vi "Sequencer.201812.vi"() -> ()   [LabVIEW 2014]
uses:
  <vilib>/gmath/statdist.llb/Poisson Random.vi
  <vilib>/Analysis/NI_AALPro.lvlib
  <vilib>/gmath/NI_Gmath.lvlib
panel:
  in  "Ion":bool
  in  "Protect":bool
  in  "Experiment":bool
  in  "Pumping":bool
  in  "Detection":bool
  in  "Cooling":bool
  out "History":variant
  in  "Count or State":i16(ring) items=["Count", "State"]
  in  "Channel":string(combo)="c1+c2+c3+c4"
  in  "Device":string(combo)="PMT"
  in  ">":dbl=1.0
  in  "Fit":bool
  out "Peak":u32
  out "Histogram":cluster{"Axis":dbl[], "Histogram":i32[]}(graph)
  in  "Data Chapter":i16(ring) items=["All", "Detection[2]"]
  out "Average Plot":cluster{dbl, dbl}(graph)
  in  "Clear":bool
  in  "Sweep":bool
  in  "Data":bool
  out "data file":string
  in  "Sequence":string
  in  "Chapter (us)":string
  in  "Sequence File":path=path "E:/Data/Sequence/Cooling.seq"
  in  "Repeats":u32=100
  in  "Compile":bool
  in  "Send":bool
  in  "Port":refnum<visa-resource-name>="COM5"
  in  "Trigger":bool
  in  "Save":bool
  out "Item Function":refnum<vi>
  in  "Set":bool
  in  "Item":string(combo)="Time"
  out "SequenceNames":string[](array[string])
  in  "Parameter":u16(ring) items=["Cooling", "Pumping", "AWG", "Horn", "Detection[0]", "Detection[1]", "Detection[2]", "Zero"]
  in  "Scan":bool
  out "Value":dbl=1.0 format="%.4f"
  in  "Step":dbl=1.0 format="%.4f"
  in  "End":dbl=1.0 format="%.3f"
  in  "Start":dbl=1.0 format="%.3f"
  out "Counts":u32[](array[numeric])
  out "CompiledSequence":string="#DopplerCooling\r\n0.9 10100000 00000000 00000000\r\n\r\n#Pump\r\n0.3 01000000 00000000 00000000\r\n\r\n#Pulsed\r\n0.2 00100000 00000000 00000000\r\n0.4 00000100 00000000 00000000\r\n0.2 00000000 10000000 00000000\r\n0.2 01000000 00000000 01000000\n"
  out "ChapterNames":string[](array[string])
  out "ChapterPositions":u32[](array[numeric])
  out "Durations Backup":dbl[](array[numeric])
  out "Durations":dbl[](array[numeric])
  in  "Period (ns)":dbl=5.0
  out "States":string[](array[string])
  in  "Sequencer":bool
  out "Clock":string
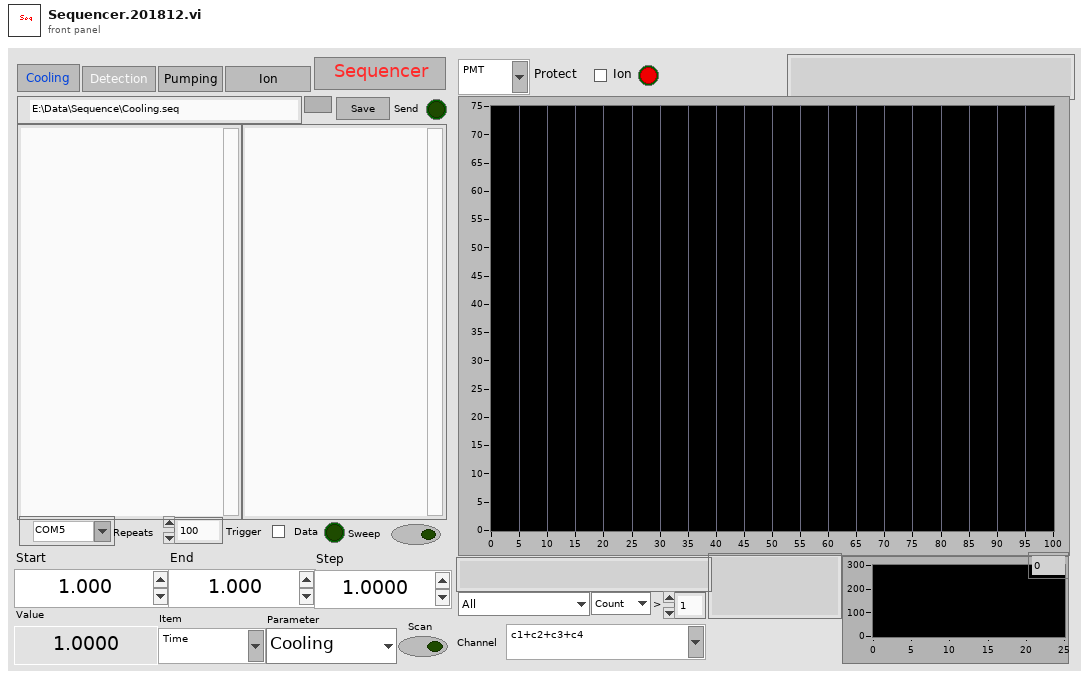
[diagram p1: front panel]
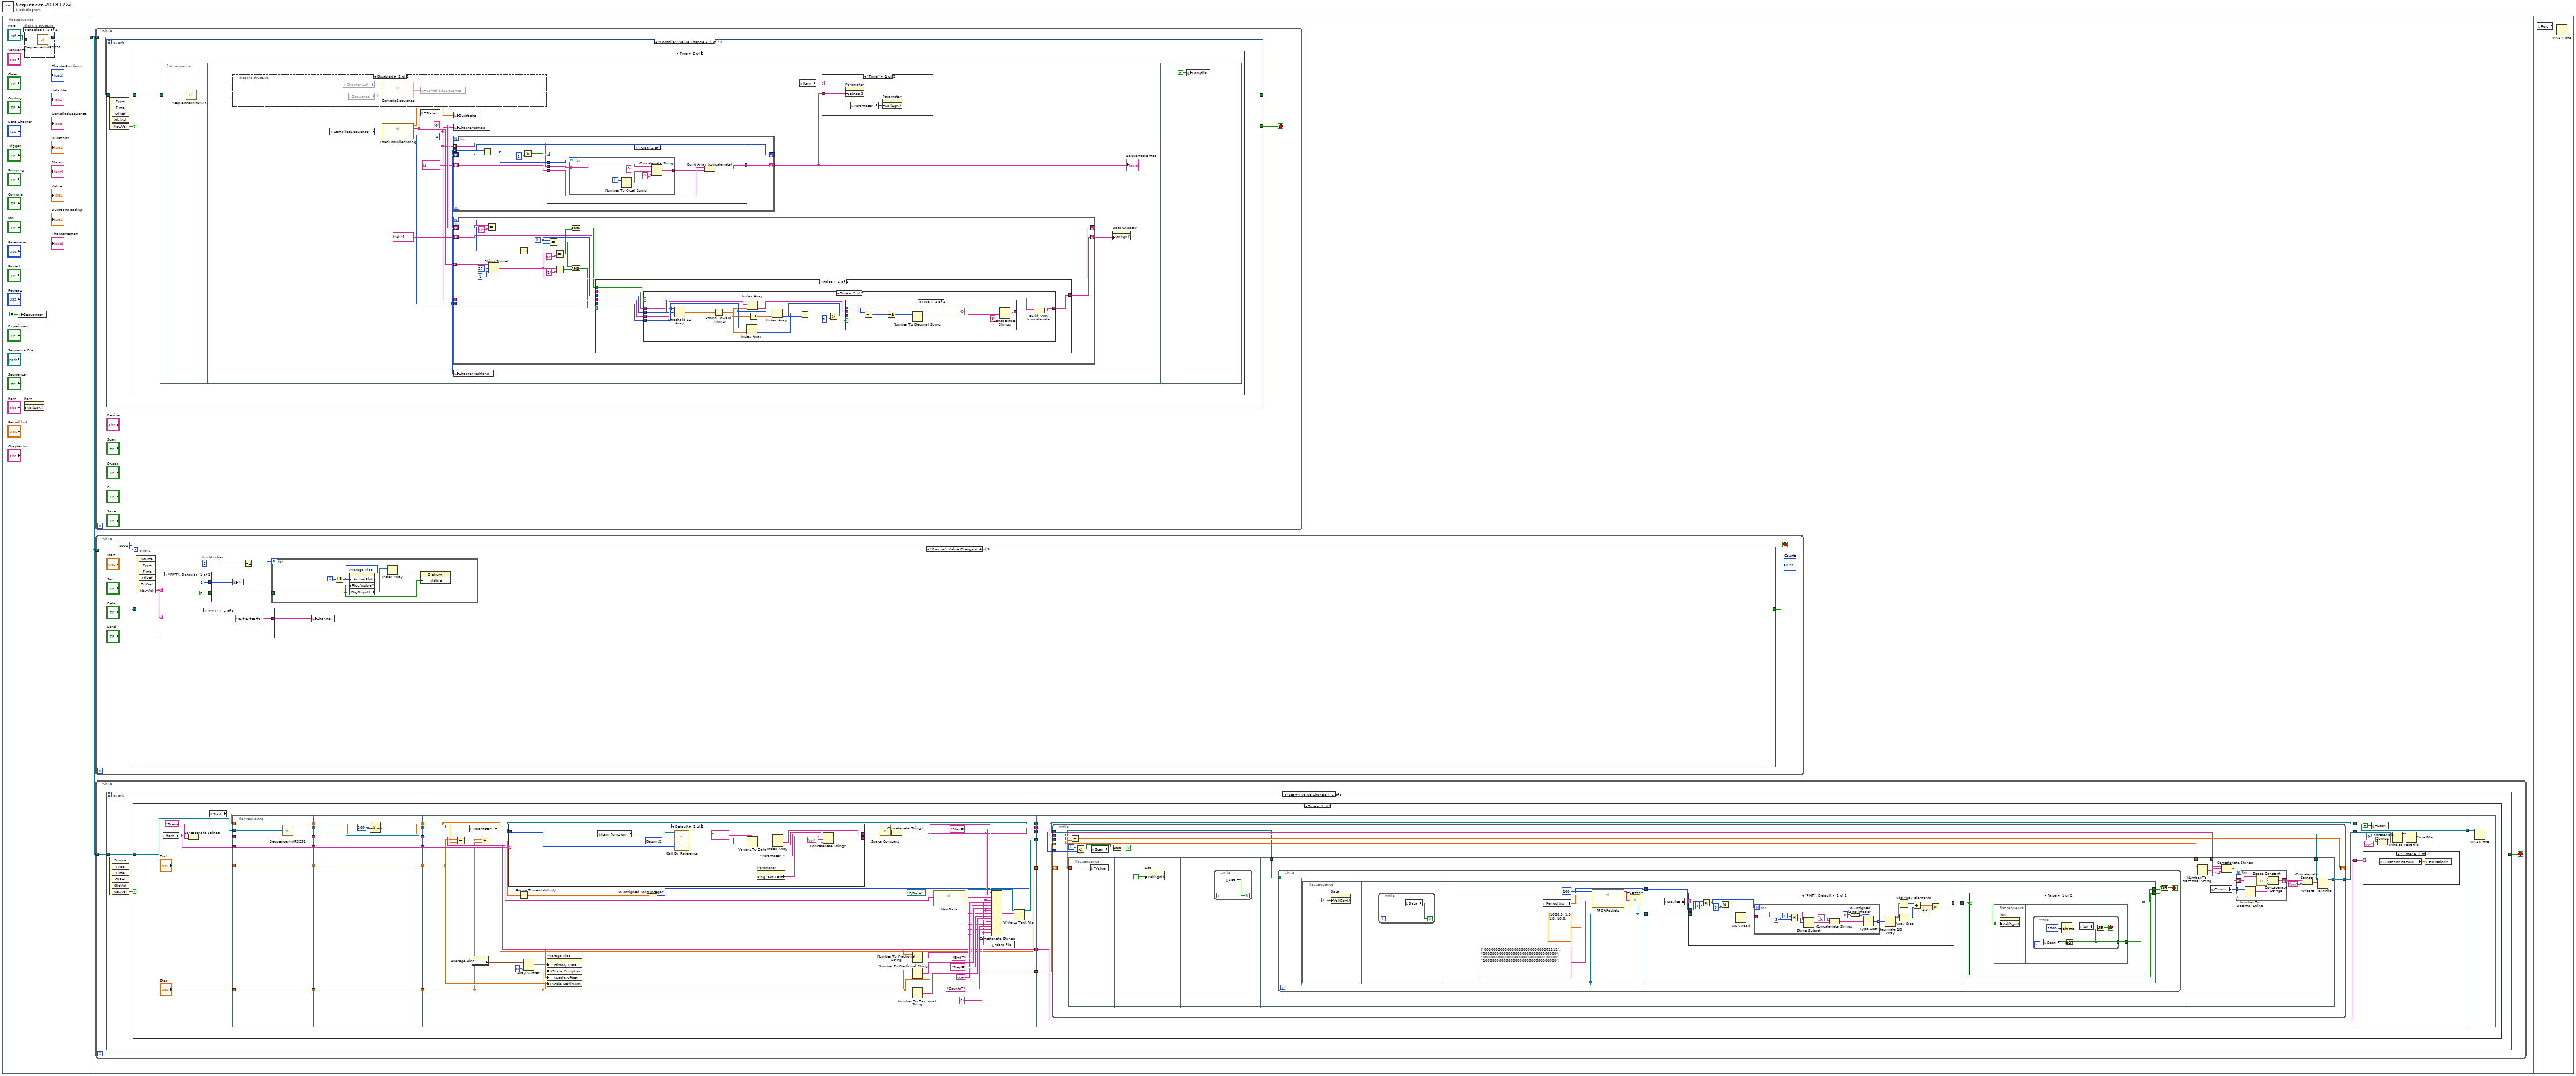
[diagram p0: block diagram]
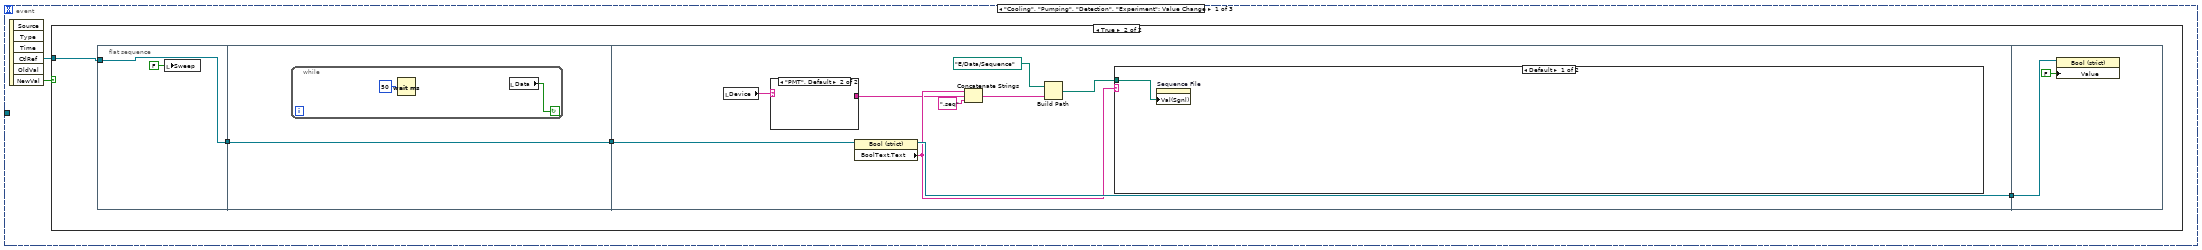
[diagram p3: hidden frame]
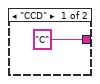
[diagram p5: hidden frame]
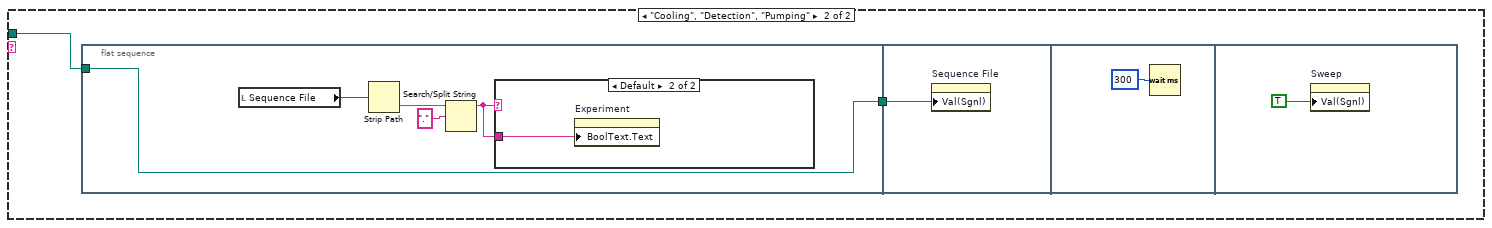
[diagram p6: hidden frame]
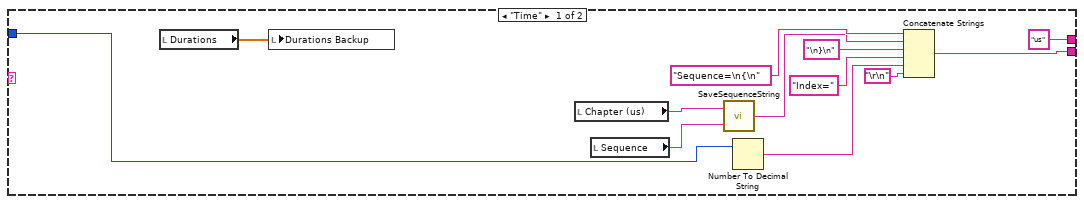
[diagram p8: hidden frame]
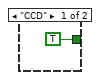
[diagram p9: hidden frame]
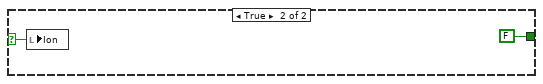
[diagram p10: hidden frame]
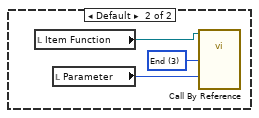
[diagram p11: hidden frame]
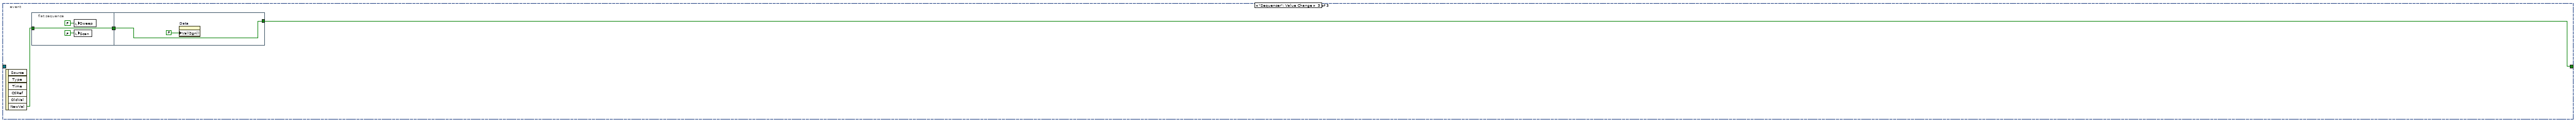
[diagram p13: hidden frame]
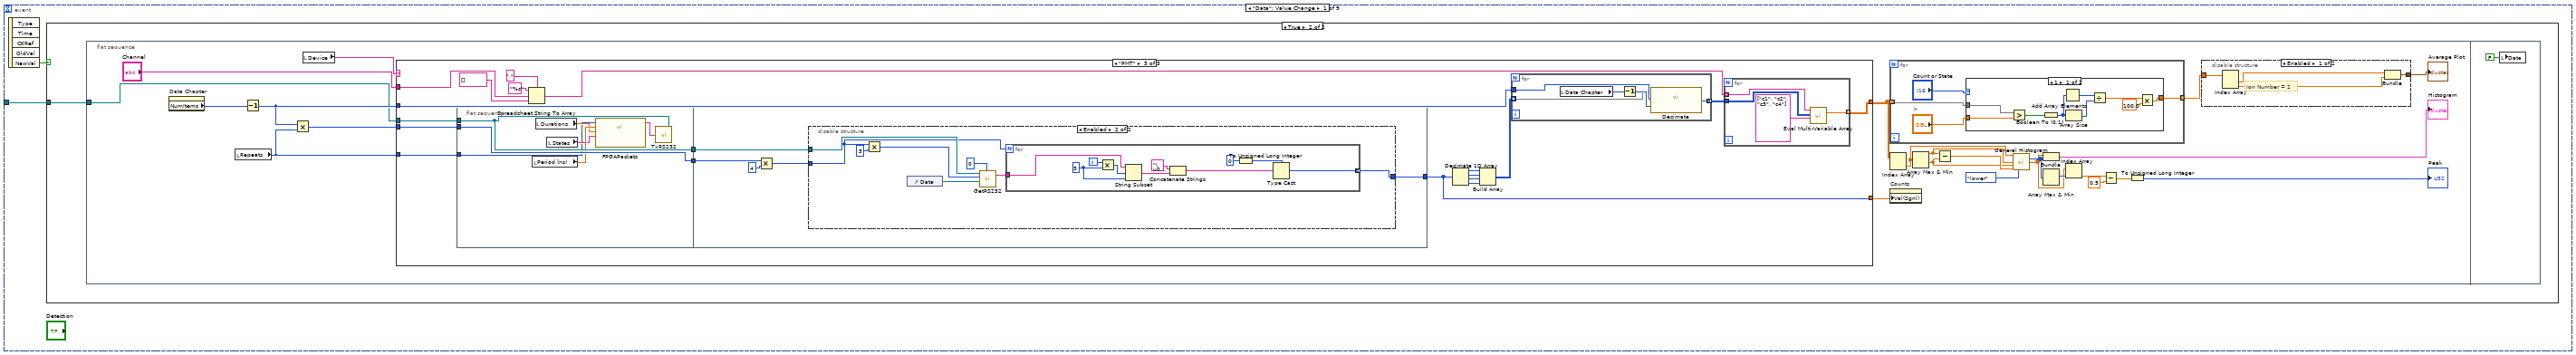
[diagram p14: hidden frame]
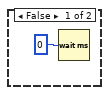
[diagram p15: hidden frame]
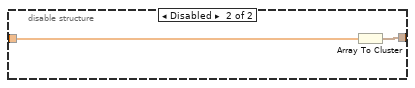
[diagram p16: hidden frame]
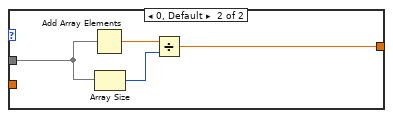
[diagram p17: hidden frame]
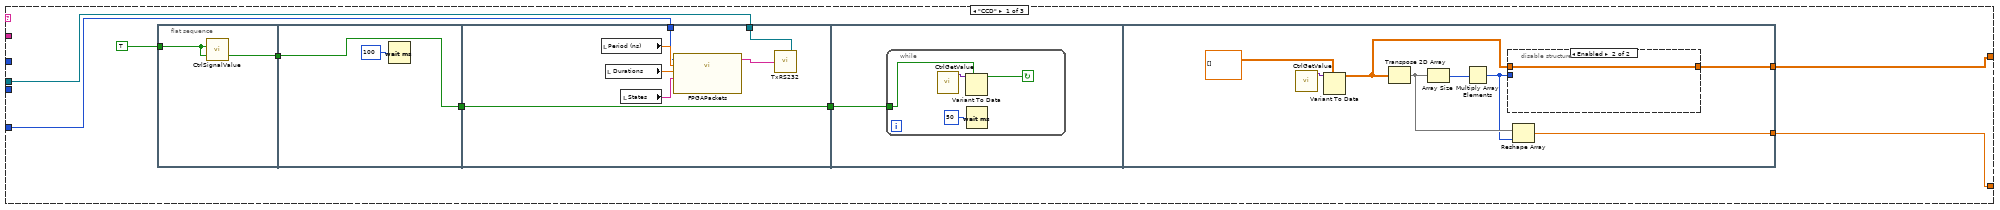
[diagram p18: hidden frame]
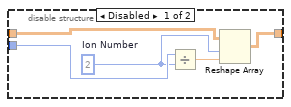
[diagram p19: hidden frame]
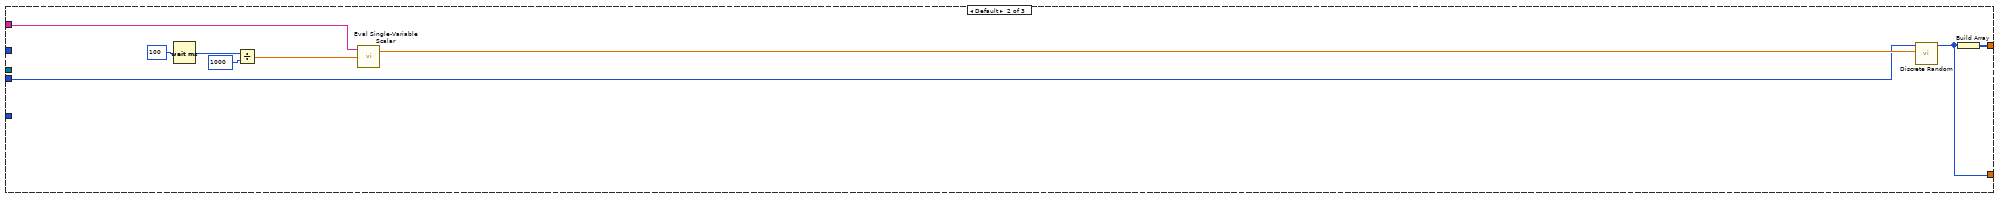
[diagram p20: hidden frame]
diagram:
  n1 = flat-sequence {
    tunnel: [w3] -> w1
    tunnel: w1 -> [w8]
    frame #0 {
      n2 = local write "Sequencer"(FALSE ("Sequencer")) -> ()
      n3 = disable-structure shown="Enabled" {
        disable-tunnel: "Port" -> [w7 _]
        disable-tunnel: [w6 _] -> w3
        frame Enabled {
          n4 = call "SequencerInitRS232.vi"("VISA resource name"=w7) -> ("reference out"=w6:refnum<visa-resource-name>)  [unwired: 1 out]
        }
        frame Disabled {
        }
      }
      n5 = property on="Item" class="CmbBox"("Val(Sgnl)"="Item") -> ()  [unwired: 2 in, 2 out]
    }
    frame #1 {
      n6 = while {
        tunnel: w8 -> [w507]
        stop <- w508 stop-if-true
        n7 = event shown="[0] \"Compile\": Value Change" {
          selector: _ -> [_ _ _ _ _ _ _ _ _ _]
          dyn-events: _ -> [_ _ _ _ _ _ _ _ _ _]
          timeout: _ -> [_ _ _ _ _ _ _ _ _ _]
          tunnel: [_ _ _ _ _ _ _ _ _ w726] -> _
          tunnel: [_ _ _ _ _ _ _ _ _ w726] -> w508
          tunnel: w507 -> [w509 _ _ _ _ _ _ _ w701 _]
          event "Compile": Value Change {
            n8 = event-data() -> ("NewVal"=w510:bool)  [unwired: 1 in, 4 out]
            n9 = case shown="True" w510 {
              tunnel: w509 -> [_ w511]
              frame False {
              }
              frame True {
                n10 = flat-sequence {
                  tunnel: w511 -> [w512]
                  frame #0 {
                    n11 = call "SequencerInitRS232.vi"("VISA resource name"=w512) -> ()  [unwired: 2 out]
                  }
                  frame #1 {
                    n12 = disable-structure shown="Disabled" {
                      frame Disabled {
                        n13 = local read "Chapter (us)"() -> (w529:string)
                        n14 = local read "Sequence"() -> (w528:string)
                        n15 = call "CompileSequence.vi"("Sequence"=w528, "Chapter"=w529) -> ("Compiled Sequence"=w527:string)
                        n16 = local write "CompiledSequence"(w527) -> ()
                      }
                      frame Enabled {
                      }
                    }
                    n17 = local read "CompiledSequence"() -> (w515:string)
                    n18 = call "LoadCompiledString.vi"("Compiled String"=w515) -> ("Durations"=w524:dbl[], "States"=w523:string[], "ChapterNames"=w516:string[], "ChapterPositions"=w517:u32[])
                    n19 = local write "States"(w523) -> ()
                    n20 = local write "Durations"(w524) -> ()
                    n21 = local write "ChapterNames"(w516) -> ()
                    n22 = for {
                      tunnel: w517 -> [w530] mode=indexing
                      tunnel: w516 -> [w531] mode=indexing
                      shift-right: [w530] -> _
                      shift-left: u32 0 ("initial scan location") -> [w537]
                      shift-right: [w532] -> w513
                      shift-left: string[] [] -> [w533]
                      n23 = Subtract(x=w530, y=w537) -> (x-y=w534:u32)
                      n24 = Greater?(x=w534, y=u32 1) -> (0:w536:bool)
                      n25 = case shown="True" w536 {
                        tunnel: w531 -> [w539 w545]
                        tunnel: w534 -> [_ w544]
                        tunnel: w533 -> [w540 w543]
                        tunnel: [w538 w541] -> w532
                        frame False {
                          n26 = Build Array (concatenate)(w540, w539) -> (w538:string[])
                        }
                        frame True {
                          n27 = for {
                            N: w544 -> [_]
                            tunnel: w545 -> [w550]
                            tunnel: [w549] -> w542 mode=indexing
                            i -> [w551]
                            n28 = Number To Octal String(2:w551) -> (0:w548:string)  [unwired: 1 in]
                            n29 = Concatenate Strings(w550, "[" ("string"), w548, "]" ("string")) -> (w549:string)
                          }
                          n30 = Build Array (concatenate)(w543, w542) -> (w541:string[])
                        }
                      }
                    }
                    "SequenceNames" <- w513
                    n31 = for {
                      N -> [w563]
                      tunnel: w523 -> [w572] mode=indexing
                      shift-right: [w560] -> _
                      shift-left: "0" -> [w570]
                      tunnel: w516 -> [w566]
                      shift-right: [w555] -> w519
                      shift-left: string[] ["All"] -> [w554]
                      tunnel: w517 -> [w553]
                      i -> [w564]
                      n32 = Equal?(x=w570, y="1") -> (x = y?=w568:bool)
                      n33 = String Subset(string=w572, offset (0)=27, length (rest)=1 ("length (rest)")) -> (substring=w560:string)
                      n34 = Decrement(x=w563) -> (x-1=w562:i32)
                      n35 = Equal?(x=w564, y=w562) -> (x = y?=w559:bool)
                      n36 = Equal?(x=w560, y="0") -> (x = y?=w565:bool)
                      n37 = Equal?(x=w560, y="1") -> (x = y?=w558:bool)
                      n38 = And(x=w568, y=w565) -> (x .and. y?=w556:bool)
                      n39 = And(x=w559, y=w558) -> (x .and. y?=w557:bool)
                      n40 = case shown="False" w557 {
                        tunnel: w566 -> [w578 w618]
                        tunnel: w554 -> [w577 w620]
                        tunnel: w564 -> [w576 _]
                        tunnel: w556 -> [w575 _]
                        tunnel: [w574 w619] -> w555
                        tunnel: w553 -> [w573 w612]
                        frame False {
                          n41 = case shown="True" w575 {
                            tunnel: w576 -> [_ w590]
                            tunnel: w578 -> [_ w591]
                            tunnel: w577 -> [w579 w593]
                            tunnel: [w579 w594] -> w574
                            tunnel: w573 -> [_ w587]
                            frame False {
                            }
                            frame True {
                              n42 = Threshold 1D Array(2:w590, 3:w587) -> (0:w592:dbl)  [unwired: 1 in]
                              n43 = Round Toward +Infinity(x=w592) -> (ceil(x): smallest int >= x=w585:dbl)
                              n44 = Index Array(array=w587, index=w585) -> (element=w584:u32)
                              n45 = Index Array(array=w591, index=w585) -> (element=w588:string)
                              n46 = Decrement(x=w585) -> (x-1=w586:dbl)
                              n47 = Index Array(array=w587, index=w586) -> (element=w580:u32)
                              n48 = Subtract(x=w584, y=w580) -> (x-y=w583:u32)
                              n49 = Greater?(x=w583, y=u32 1) -> (0:w581:bool)
                              n50 = case shown="True" w581 {
                                tunnel: w590 -> [_ w604]
                                tunnel: [w595 w598] -> w589
                                tunnel: w588 -> [w595 w597]
                                tunnel: w580 -> [_ w596]
                                frame False {
                                }
                                frame True {
                                n51 = Subtract(x=w604, y=w596) -> (x-y=w603:u32)
                                n52 = Decrement(x=w603) -> (x-1=w602:u32)
                                n53 = Number To Decimal String(number=w602) -> (decimal integer string=w599:string)  [unwired: 1 in]
                                n54 = Concatenate Strings(w597, "[" ("element"), w599, "]" ("element")) -> (w598:string)
                                }
                              }
                              n55 = Build Array (concatenate)(w593, w589) -> (w594:string[])
                            }
                          }
                        }
                        frame True {
                          n56 = Array Size(array=w618) -> (size(s)=w617:i32)
                          n57 = Array Size(array=w612) -> (size(s)=w615:i32)
                          n58 = Decrement(x=w617) -> (x-1=w616:i32)
                          n59 = Decrement(x=w615) -> (x-1=w614:i32)
                          n60 = Index Array(array=w612, index=w614) -> (element=w611:u32)
                          n61 = Index Array(array=w618, index=w616) -> (element=w607:string)
                          n62 = Decrement(x=w614) -> (x-1=w613:i32)
                          n63 = Index Array(array=w612, index=w613) -> (element=w610:u32)
                          n64 = Subtract(x=w611, y=w610) -> (x-y=w605:u32)
                          n65 = Greater?(x=w605, y=u32 1) -> (0:w608:bool)
                          n66 = case shown="True" w608 {
                            tunnel: w607 -> [w621 w628]
                            tunnel: [w621 w622] -> w606
                            tunnel: w605 -> [_ w625]
                            frame False {
                            }
                            frame True {
                              n67 = Decrement(x=w625) -> (x-1=w624:u32)
                              n68 = Number To Octal String(2:w624) -> (0:w623:string)  [unwired: 1 in]
                              n69 = Concatenate Strings(w628, "[" ("string"), w623, "]" ("string")) -> (w622:string)
                            }
                          }
                          n70 = Build Array (concatenate)(w620, w606) -> (w619:string[])
                        }
                      }
                    }
                    n71 = local write "ChapterPositions"(w517) -> ()
                    n72 = local read "Item"() -> (w514:string)
                    n73 = case shown="\"Time\"" w514 {
                      tunnel: w513 -> [w526 _]
                      frame "Time" {
                        n74 = property on="Parameter" class="Ring (strict)"("Strings []"=w526) -> ()  [unwired: 2 in, 2 out]
                        n75 = local read "Parameter"() -> (w525:u16)
                        n76 = property on="Parameter" class="Ring (strict)"("Val(Sgnl)"=w525) -> ()  [unwired: 2 in, 2 out]
                      }
                      frame Default {
                      }
                    }
                    n77 = property on="Data Chapter" class="Ring (strict)"("Strings []"=w519) -> ()  [unwired: 2 in, 2 out]
                  }
                  frame #2 {
                    n78 = local write "Compile"(FALSE ("Compile")) -> ()
                  }
                }
              }
            }
          }
          event "Item": Value Change {
            n79 = event-data() -> ("NewVal"=w631:string)  [unwired: 1 in, 5 out]
            n80 = flat-sequence {
              tunnel: w631 -> [w635]
              tunnel: [w635] -> w630
              tunnel: w630 -> [w637]
              frame #0 {
                w634 = u32 1 items=["Open", "Close", "Begin", "End", "Get", "Set"] ("Mode")
                n81 = local read "Item Function"() -> (w633:refnum<vi>)
                n82 = call-by-ref "?"(reference=w633, "Mode"=w634) -> (error out=w632:errorcluster)  [unwired: 2 in, 2 out]
                n83 = call <vilib>:"Clear Errors.vi"("error in (no error)"=w632) -> ()  [unwired: 5 in, 2 out]
              }
              frame #1 {
                n84 = case shown="Default" w637 {
                  selector: w637 -> [w645 _]
                  tunnel: [w638 w650] -> w636
                  frame Default {
                    w641 = u32 0 items=["Open", "Close", "Begin", "End", "Get", "Set"] ("Mode")
                    n85 = Concatenate Strings(w645, ".vi" ("string")) -> (w643:string)
                    n86 = Current VI's Path() -> (path=w647:path)
                    n87 = Strip Path(path=w647) -> (stripped path=w646:path)  [unwired: 1 out]
                    n88 = Build Path(base path=w646, name or relative path=w643) -> (appended path=w648:path)
                    n89 = Open VI Reference(type specifier VI Refnum (for type only)=refnum<vi> refnum, vi path=w648) -> (vi reference=w642:refnum<vi>)  [unwired: 4 in, 1 out]
                    "Item Function" <- w642
                    n90 = call-by-ref "?"(reference=w642, "Mode"=w641) -> ("Out"=w640:variant)  [unwired: 2 in, 2 out]
                    n91 = Variant To Data(type=string[] [] ("Strings []"), Variant=w640) -> (data=w638:string[])  [unwired: 1 in, 1 out]
                  }
                  frame "Time" {
                    n92 = local read "SequenceNames"() -> (w650:string[])
                  }
                }
                n93 = property on="Parameter" class="Ring (strict)"("Strings []"=w636) -> ()  [unwired: 2 in, 2 out]
              }
              frame #2 {
                n94 = disable-structure shown="Enabled" {
                  disable-tunnel: [w652 u16 0 ("Parameter")] -> w651
                  frame Disabled {
                    n95 = local read "Parameter"() -> (w652:u16)
                  }
                  frame Enabled {
                  }
                }
                n96 = property on="Parameter" class="Ring (strict)"("Val(Sgnl)"=w651) -> ()  [unwired: 2 in, 2 out]
              }
            }
          }
          event "Parameter": Value Change {
            n97 = event-data() -> ("NewVal"=w654:u16)  [unwired: 1 in, 5 out]
            n98 = local read "Item"() -> (w656:string)
            n99 = case shown="Default" w656 {
              tunnel: [w658 w661] -> w655
              tunnel: w654 -> [w657 w660]
              frame "Time" {
                n100 = local read "Durations"() -> (w659:dbl[])
                n101 = Index Array(array=w659, index=w657) -> (element=w658:dbl)
              }
              frame Default {
                w664 = u32 4 items=["Open", "Close", "Begin", "End", "Get", "Set"] ("Mode")
                n102 = local read "Item Function"() -> (w665:refnum<vi>)
                n103 = call-by-ref "?"(reference=w665, "In"=w660, "Mode"=w664) -> ("Out"=w663:variant)  [unwired: 1 in, 2 out]
                n104 = Variant To Data(type=0.0, Variant=w663) -> (data=w661:dbl)  [unwired: 1 in, 1 out]
              }
            }
            n105 = local write "Value"(w655) -> ()
          }
          event "Save": Value Change {
            n106 = event-data() -> ("NewVal"=w666:bool)  [unwired: 1 in, 4 out]
            n107 = case shown="True" w666 {
              frame False {
              }
              frame True {
                n108 = flat-sequence {
                  frame #0 {
                    n109 = local read "Sequence File"() -> (w671:path)
                    n110 = local read "Chapter (us)"() -> (w669:string)
                    n111 = local read "Sequence"() -> (w668:string)
                    n112 = call "SaveSequenceString.vi"("Sequence"=w668, "Chapter"=w669) -> ("Sequence String"=w670:string)
                    n113 = call "CompileSequence.vi"("Sequence"=w668, "Chapter"=w669) -> ("Compiled Sequence"=w667:string)
                    n114 = Not Equal?(x=w671, y=path "") -> (x != y?=w673:bool)
                    n115 = case shown="True" w673 {
                      tunnel: w671 -> [_ w675]
                      tunnel: w670 -> [_ w674]
                      frame False {
                      }
                      frame True {
                        n116 = Write to Text File(file (use dialog)=w675, text=w674) -> ()  [unwired: 2 in, 3 out]
                      }
                    }
                    n117 = local write "CompiledSequence"(w667) -> ()
                  }
                  frame #1 {
                    n118 = local write "Save"(FALSE ("Compile")) -> ()
                    n119 = property on="Compile" class="Bool (strict)"("Val(Sgnl)"=TRUE ("Value (Signaling)")) -> ()  [unwired: 2 in, 2 out]
                  }
                }
              }
            }
          }
          event "Fit": Value Change {
            n120 = event-data() -> ("NewVal"=w678:bool)  [unwired: 1 in, 4 out]
            n121 = case shown="True" w678 {
              frame False {
              }
              frame True {
                n122 = local write "Fit"(FALSE ("Fit")) -> ()
                n123 = property on="Average Plot" class="WFChart (strict)"() -> ("History Data"=w680:cluster{dbl, dbl}[])  [unwired: 2 in, 2 out]
                n124 = To Variant(anything=w680) -> (Variant=→"History":variant)
              }
            }
          }
          event "Clear": Value Change {
            n125 = event-data() -> ()  [unwired: 1 in, 6 out]
            n126 = property on="Average Plot" class="WFChart (strict)"() -> ("History Data"=w684:cluster{dbl, dbl}[])  [unwired: 2 in, 2 out]
            n127 = Array Subset(array=w684, length=0) -> (w683:cluster{dbl, dbl}[])  [unwired: 1 in]
            n128 = property on="Average Plot" class="WFChart (strict)"("History Data"=w683) -> ()  [unwired: 2 in, 2 out]
          }
          event "Sequence File": Value Change {
            n129 = event-data() -> ("NewVal"=w686:path)  [unwired: 1 in, 4 out]
            n130 = call <vilib>:"Check if File or Folder Exists.vi"("path"=w686) -> ("file or folder exists?"=w687:bool, "dup path"=w685:path)  [unwired: 8 in, 1 out]
            n131 = case shown="True" w687 {
              tunnel: w685 -> [_ w688]
              frame False {
              }
              frame True {
                n132 = flat-sequence {
                  tunnel: w688 -> [w692]
                  frame #0 {
                    n133 = Read from Text File(file (use dialog)=w692) -> (text=w693:string)  [unwired: 3 in, 3 out]
                    n134 = call "LoadSequenceString.vi"("Sequence String"=w693) -> ("Chapter"=w691:string, "Sequence"=w690:string)
                    n135 = local write "Chapter (us)"(w691) -> ()
                    n136 = call "CompileSequence.vi"("Sequence"=w690, "Chapter"=w691) -> ("Compiled Sequence"=w689:string)
                    n137 = local write "Sequence"(w690) -> ()
                    n138 = local write "CompiledSequence"(w689) -> ()
                  }
                  frame #1 {
                    n139 = property on="Compile" class="Bool (strict)"("Val(Sgnl)"=TRUE ("Value (Signaling)")) -> ()  [unwired: 2 in, 2 out]
                  }
                }
              }
            }
          }
          event "Repeats": Value Change {
            n140 = event-data() -> ("NewVal"=w696:u32)  [unwired: 1 in, 5 out]
            n141 = local read "Device"() -> (w695:string)
            n142 = case shown="\"CCD\"" w695 {
              tunnel: w696 -> [_ w698]
              frame "PMT", Default {
              }
              frame "CCD" {
                n143 = property on="Data Chapter" class="Ring (strict)"() -> ("NumItems"=w700:u32)  [unwired: 2 in, 2 out]
                n144 = Decrement(x=w700) -> (x-1=w699:u32)
                n145 = Multiply(x=w699, y=w698) -> (x*y=w697:u32)
                n146 = call "CtrlSignalValue.vi"("variant"=w697) -> ()  [unwired: 3 in, 1 out]
              }
            }
          }
          event "Sweep": Value Change {
            n147 = event-data() -> ("NewVal"=w702:bool)  [unwired: 1 in, 4 out]
            n148 = case shown="True" w702 {
              tunnel: w701 -> [_ w707]
              frame False {
              }
              frame True {
                n149 = flat-sequence {
                  tunnel: w707 -> [w709]
                  tunnel: [w708] -> w704
                  tunnel: w704 -> [w711]
                  tunnel: [w711] -> w703
                  tunnel: [w712] -> w706
                  tunnel: w703 -> [w712]
                  tunnel: w706 -> [w721]
                  tunnel: [w721] -> w705
                  tunnel: w705 -> [w725]
                  frame #0 {
                    n150 = call "SequencerInitRS232.vi"("VISA resource name"=w709) -> ("reference out"=w708:refnum<visa-resource-name>)  [unwired: 1 out]
                  }
                  frame #1 {
                    n151 = Wait (ms)(milliseconds to wait=u32 200) -> ()  [unwired: 1 out]
                  }
                  frame #2 {
                    n152 = local write "data file"("") -> ()
                    n153 = property on="Average Plot" class="WFChart (strict)"() -> ("History Data"=w715:cluster{dbl, dbl}[])  [unwired: 2 in, 2 out]
                    n154 = Array Subset(array=w715, length=0) -> (w713:cluster{dbl, dbl}[])  [unwired: 1 in]
                    n155 = property on="Average Plot" class="WFChart (strict)"("History Data"=w713) -> (error out=w717:errorcluster)  [unwired: 2 in, 1 out]
                    n156 = property on="Average Plot" class="WFChart (strict)"(error in=w717, "XScale.Multiplier"=1.0 ("X Scale.Offset and Multiplier:Multiplier"), "XScale.Offset"=0.0 ("X Scale.Offset and Multiplier:Offset"), "XScale.Maximum"=100.0 ("X Scale.Range:Maximum")) -> ()  [unwired: 1 in, 2 out]
                  }
                  frame #3 {
                    n157 = while {
                      stop <- w722 continue-if-true
                      n158 = flat-sequence {
                        frame #0 {
                          n159 = property on="Data" class="Bool (strict)"("Val(Sgnl)"=TRUE ("Value (Signaling)")) -> ()  [unwired: 2 in, 2 out]
                        }
                        frame #1 {
                          n160 = while {
                            stop <- w724 continue-if-true
                            n161 = local read "Data"() -> (w724:bool)
                          }
                        }
                      }
                      n162 = local read "Sweep"() -> (w722:bool)
                    }
                  }
                  frame #4 {
                    n163 = VISA Close(VISA resource name=w725) -> ()  [unwired: 1 in, 1 out]
                  }
                }
              }
            }
          }
          event "Sequencer": Value Change {
            n164 = event-data() -> ("NewVal"=w726:bool)  [unwired: 1 in, 4 out]
          }
        }
      }
      n165 = while {
        tunnel: w8 -> [w268]
        stop <- w267 stop-if-true
        n166 = event shown="[3] \"Device\": Value Change" {
          selector: _ -> [_ _ _ _ _ _ _ _ _]
          dyn-events: _ -> [_ _ _ _ _ _ _ _ _]
          timeout: u32 1000 ("milliseconds to wait") -> [_ _ _ _ _ _ _ _ _]
          tunnel: w268 -> [w270 _ _ _ _ _ _ _ w497]
          tunnel: [_ _ _ _ _ _ _ w496 _] -> w267
          event "Data": Value Change {
            n167 = event-data() -> ("NewVal"=w269:bool)  [unwired: 1 in, 4 out]
            n168 = case shown="True" w269 {
              tunnel: w270 -> [_ w272]
              frame False {
                n169 = Wait (ms)(milliseconds to wait=u32 0) -> ()  [unwired: 1 out]
              }
              frame True {
                n170 = flat-sequence {
                  tunnel: w272 -> [w295]
                  frame #0 {
                    n171 = property on="Data Chapter" class="Ring (strict)"() -> ("NumItems"=w294:u32)  [unwired: 2 in, 2 out]
                    n172 = local read "Repeats"() -> (w273:u32)
                    n173 = Decrement(x=w294) -> (x-1=w296:u32)
                    n174 = Multiply(x=w296, y=w273) -> (x*y=w293:u32)
                    n175 = local read "Device"() -> (w274:string)
                    n176 = case shown="\"PMT\"" w274 {
                      tunnel: w296 -> [_ _ w377]
                      tunnel: w295 -> [w323 _ w384]
                      tunnel: w293 -> [_ w364 w383]
                      tunnel: [w325 w363 w382] -> w282
                      tunnel: [w326 w362 w374] -> w276
                      tunnel: "Channel" -> [_ w357 w369]
                      tunnel: w273 -> [w320 _ w366]
                      frame "CCD" {
                        n177 = flat-sequence {
                          tunnel: TRUE -> [w328]
                          tunnel: [w328] -> w322
                          tunnel: w322 -> [w330]
                          tunnel: [w330] -> w321
                          tunnel: w321 -> [w337]
                          tunnel: [w337] -> w324
                          tunnel: w323 -> [w336]
                          tunnel: w320 -> [w331]
                          tunnel: w324 -> [w338]
                          tunnel: [w345] -> w326
                          tunnel: [w347] -> w325
                          frame #0 {
                            n178 = call "CtrlSignalValue.vi"("variant"=w328) -> ()  [unwired: 3 in, 1 out]
                          }
                          frame #1 {
                            n179 = Wait (ms)(milliseconds to wait=u32 100) -> ()  [unwired: 1 out]
                          }
                          frame #2 {
                            n180 = local read "Period (ns)"() -> (w334:dbl)
                            n181 = local read "Durations"() -> (w333:dbl[])
                            n182 = local read "States"() -> (w332:string[])
                            n183 = call "FPGAPackets.vi"("Repeats"=w331, "Period (ns)"=w334, "Durations"=w333, "States"=w332) -> ("Packets"=w335:string)  [unwired: 1 in, 1 out]
                            n184 = call "TxRS232.vi"("VISA resource name"=w336, "Data"=w335) -> ()
                          }
                          frame #3 {
                            n185 = while {
                              tunnel: w338 -> [w340]
                              stop <- w339 continue-if-true
                              n186 = call "CtrlGetValue.vi"() -> ("variant"=w342:variant)  [unwired: 2 in, 3 out]
                              n187 = Variant To Data(type=w340, Variant=w342) -> (data=w339:bool)  [unwired: 1 in, 1 out]
                              n188 = Wait (ms)(milliseconds to wait=u32 50) -> ()  [unwired: 1 out]
                            }
                          }
                          frame #4 {
                            n189 = call "CtrlGetValue.vi"() -> ("variant"=w350:variant)  [unwired: 2 in, 3 out]
                            n190 = Variant To Data(type=dbl[][] [] ("Count"), Variant=w350) -> (data=w343:dbl[][])  [unwired: 1 in, 1 out]
                            n191 = Transpose 2D Array(2D array=w343) -> (transposed array=w346:dbl[][])
                            n192 = Array Size(array=w346) -> (size(s)=w348:i32[])
                            n193 = Multiply Array Elements(1:w348) -> (0:w344:i32)
                            n194 = disable-structure shown="Enabled" {
                              disable-tunnel: [w355 w356] -> w345
                              disable-tunnel: w344 -> [w354 _]
                              disable-tunnel: w343 -> [w351 w356]
                              frame Disabled {
                                w353 = 2  # Ion Number
                                n195 = Divide(x=w354, y=w353) -> (x/y=w352:dbl)
                                n196 = Reshape Array(w351, w353, w352) -> (w355:dbl[][])
                              }
                              frame Enabled {
                              }
                            }
                            n197 = Reshape Array(w346, w344) -> (w347:dbl[])
                          }
                        }
                      }
                      frame Default {
                        n198 = Wait (ms)(milliseconds to wait=u32 100 ("y")) -> (millisecond timer value=w359:u32)
                        n199 = Divide(x=w359, y=u32 1000) -> (x/y=w361:dbl)
                        n200 = call <vilib>:"Eval Single-Variable Scalar.vi"("x value"=w361, "formula"=w357) -> ("y value"=w365:dbl)  [unwired: 1 in, 1 out]
                        n201 = call-poly <vilib>:"Discrete Random.vi"("lambda"=w365, "samples"=w364) -> ("Poisson random data"=w363:i32[])  [unwired: 8 in, 1 out]
                        n202 = Build Array(w363) -> (w362:i32[][])
                      }
                      frame "PMT" {
                        n203 = flat-sequence {
                          tunnel: w383 -> [w391]
                          tunnel: w384 -> [w390]
                          tunnel: [w390] -> w368
                          tunnel: [w391] -> w367
                          tunnel: w366 -> [w385]
                          tunnel: [w392] -> w382
                          tunnel: w368 -> [w396]
                          tunnel: w367 -> [w395]
                          frame #0 {
                            n204 = local read "Period (ns)"() -> (w388:dbl)
                            n205 = local read "Durations"() -> (w387:dbl[])
                            n206 = local read "States"() -> (w386:string[])
                            n207 = call "FPGAPackets.vi"("Repeats"=w385, "Period (ns)"=w388, "Durations"=w387, "States"=w386) -> ("Packets"=w389:string)  [unwired: 1 in, 1 out]
                            n208 = call "TxRS232.vi"("VISA resource name"=w390, "Data"=w389) -> ()
                          }
                          frame #1 {
                            n209 = Multiply(x=w395, y=u32 4) -> (x*y=w394:u32)
                            n210 = disable-structure shown="Enabled" {
                              disable-tunnel: w396 -> [w399 w421]
                              disable-tunnel: w394 -> [w398 w416]
                              disable-tunnel: [w397 w417] -> w392
                              frame Disabled {
                                n211 = while {
                                tunnel: w399 -> [w411]
                                tunnel: [w412] -> w397 mode=indexing
                                tunnel: w398 -> [w409]
                                i -> [w408]
                                stop <- w414 continue-if-true
                                n212 = Increment(x=w408) -> (x+1=w407:i32)
                                n213 = control-ref of="Data"() -> (w410:refnum<vi>)
                                n214 = Less?(x=w407, y=w409) -> (x < y?=w413:bool)
                                n215 = local read "Data"() -> (w415:bool)
                                n216 = And(x=w413, y=w415) -> (x .and. y?=w414:bool)
                                n217 = call "GetRS232.vi"("VISA resource name"=w411, "Bytes To Read"=3, "Control"=w410, "Limit"=0) -> ("Data"=w401:string)  [unwired: 1 in, 1 out]
                                n218 = Concatenate Strings("\u0000" ("string"), w401) -> (w403:string)
                                n219 = To Unsigned Long Integer(number=u32 0) -> (unsigned 32bit integer=w406:u32)
                                n220 = Type Cast(type=w406, x=w403) -> (*(type *) &x=w412:u32)
                                }
                              }
                              frame Enabled {
                                n221 = Multiply(x=w416, y=3 ("Bytes To Read")) -> (x*y=w420:u32)
                                n222 = control-ref of="Data"() -> (w419:refnum<vi>)
                                n223 = call "GetRS232.vi"("VISA resource name"=w421, "Bytes To Read"=w420, "Control"=w419, "Limit"=0) -> ("Data"=w418:string)  [unwired: 1 in, 1 out]
                                n224 = for {
                                N: w416 -> [_]
                                tunnel: w418 -> [w433]
                                tunnel: [w424] -> w417 mode=indexing
                                i -> [w427]
                                w426 = 3 ("length (rest)")
                                n225 = Multiply(x=w427, y=w426) -> (x*y=w425:i32)
                                n226 = String Subset(string=w433, offset (0)=w425, length (rest)=w426) -> (substring=w428:string)
                                n227 = Concatenate Strings("\u0000" ("string"), w428) -> (w432:string)
                                n228 = To Unsigned Long Integer(number=u32 0) -> (unsigned 32bit integer=w429:u32)
                                n229 = Type Cast(type=w429, x=w432) -> (*(type *) &x=w424:u32)
                                }
                              }
                            }
                          }
                        }
                        n230 = Spreadsheet String To Array(delimiter (Tab)=",", format string="%s", spreadsheet string=w369, array type (2D Dbl)=string[] []) -> (array=w370:string[])
                        n231 = Decimate 1D Array(w382) -> (w381:u32[], w380:u32[], w379:u32[], w378:u32[])
                        n232 = Build Array(w381, w380, w379, w378) -> (w376:u32[][])
                        n233 = for {
                          tunnel: w377 -> [w436]
                          tunnel: w376 -> [w435] mode=indexing
                          tunnel: [w434] -> w375 mode=indexing
                          n234 = local read "Data Chapter"() -> (w437:i16)
                          n235 = Decrement(x=w437) -> (x-1=w438:i16)
                          n236 = call "Decimate.vi"("i"=w438, "n"=w436, "Input Array"=w435) -> ("Decimated Array"=w434:u32[])
                        }
                        n237 = for {
                          tunnel: w375 -> [w442]
                          tunnel: [w440] -> w374 mode=indexing
                          tunnel: w370 -> [w439] mode=indexing
                          n238 = call <vilib>:"Eval Multi-Variable Array.vi"("Variables"=string[] ["c1", "c2", "c3", "c4"], "X Values"=w442, "formula"=w439) -> ("Y Values"=w440:dbl[])  [unwired: 1 in, 1 out]
                        }
                      }
                    }
                    n239 = for {
                      tunnel: w276 -> [w305] mode=indexing
                      tunnel: [w303] -> w279 mode=indexing
                      n240 = case shown="1" "Count or State" {
                        tunnel: [w307 w317] -> w303
                        tunnel: ">" -> [w313 _]
                        tunnel: w305 -> [w312 w316]
                        frame 1 {
                          n241 = Greater?(x=w312, y=w313) -> (0:w314:bool[])
                          n242 = Boolean To (0,1)(Boolean=w314) -> (0, 1=w309:i16[])
                          n243 = Add Array Elements(numeric array=w309) -> (sum=w310:i16)
                          n244 = Array Size(array=w309) -> (size(s)=w311:i32)
                          n245 = Divide(x=w310, y=w311) -> (x/y=w308:dbl)
                          n246 = Multiply(x=w308, y=100.0) -> (x*y=w307:dbl)
                        }
                        frame 0, Default {
                          n247 = Add Array Elements(numeric array=w316) -> (sum=w318:dbl)
                          n248 = Array Size(array=w316) -> (size(s)=w319:i32)
                          n249 = Divide(x=w318, y=w319) -> (x/y=w317:dbl)
                        }
                      }
                    }
                    n250 = Index Array(array=w276) -> (element=w277:dbl[])  [unwired: 2 in]
                    n251 = property on="Counts" class="Arr (strict)"("Val(Sgnl)"=w282) -> ()  [unwired: 2 in, 2 out]
                    n252 = Array Max & Min(array=w277) -> (max value=w291:dbl, min value=w289:dbl)  [unwired: 2 out]
                    n253 = Subtract(x=w291, y=w289) -> (x-y=w290:dbl)
                    n254 = call <vilib>:"General Histogram.vi"("X"=w277, "max"=w291, "min"=w289, "# bins"=w290, "inclusion"=enum32{"lower", "upper"}."lower") -> ("Histogram"=w288:i32[], "Axis"=w286:dbl[])  [unwired: 6 in, 3 out]
                    n255 = Bundle("Axis"=w286, "Histogram"=w288) -> (→"Histogram":cluster{"Axis":dbl[], "Histogram":i32[]})  [unwired: 1 in]
                    n256 = Array Max & Min(array=w288) -> (max index (indices)=w287:i32)  [unwired: 3 out]
                    n257 = Index Array(array=w286, index=w287) -> (element=w284:dbl)
                    n258 = Subtract(x=w284, y=0.5) -> (x-y=w280:dbl)
                    n259 = To Unsigned Long Integer(number=w280) -> (unsigned 32bit integer=→"Peak":u32)
                    n260 = disable-structure shown="Enabled" {
                      disable-tunnel: w279 -> [w299 w302]
                      disable-tunnel: [w298 w301] -> w278
                      frame Enabled {
                        # "Ion Number = 2"
                        n261 = Index Array(array=w299) -> (element #1=w300:dbl, element #2=w297:dbl)  [unwired: 2 in]
                        n262 = Bundle(w300, w297) -> (w298:cluster{dbl, dbl})  [unwired: 1 in]
                      }
                      frame Disabled {
                        n263 = Array To Cluster(array=w302) -> (cluster=w301:cluster{"[0]":dbl, "[1]":dbl})
                      }
                    }
                    "Average Plot" <- w278
                  }
                  frame #1 {
                    n264 = local write "Data"(FALSE ("Acquisition")) -> ()
                  }
                }
              }
            }
          }
          event "Ion": Value Change {
            n265 = event-data() -> ("NewVal"=w444:bool)  [unwired: 1 in, 5 out]
            n266 = case shown="False" w444 {
              frame False {
                n267 = local read "Protect"() -> (w445:bool)
                n268 = case shown="True" w445 {
                  frame False {
                  }
                  frame True {
                    n269 = flat-sequence {
                      frame #0 {
                        n270 = local read "Sequence File"() -> (w449:path)
                        n271 = Strip Path(path=w449) -> (name=w448:string)  [unwired: 1 out]
                        n272 = Search/Split String(string=w448, search string/char (-)=".") -> (substring before match=w446:string)  [unwired: 1 in, 2 out]
                        n273 = property on="Experiment" class="Bool (strict)"("BoolText.Text"=w446) -> ()  [unwired: 2 in, 2 out]
                      }
                      frame #1 {
                        n274 = Build Path(base path=path "E:/Data/Sequence", name or relative path="Ion.seq" ("string")) -> (appended path=w451:path)
                        n275 = property on="Sequence File" class="Path"("Val(Sgnl)"=w451) -> ()  [unwired: 2 in, 2 out]
                      }
                      frame #2 {
                        n276 = Wait (ms)(milliseconds to wait=u32 300) -> ()  [unwired: 1 out]
                      }
                      frame #3 {
                        n277 = property on="Sweep" class="Bool (strict)"("Val(Sgnl)"=TRUE ("Value (Signaling)")) -> ()  [unwired: 2 in, 2 out]
                      }
                    }
                  }
                }
              }
              frame True {
              }
            }
          }
          event "Set": Value Change {
            n278 = event-data() -> ("NewVal"=w455:bool)  [unwired: 1 in, 5 out]
            n279 = case shown="True" w455 {
              frame False {
              }
              frame True {
                n280 = flat-sequence {
                  frame #0 {
                    n281 = local read "Value"() -> (w456:dbl)
                    n282 = local read "Item"() -> (w457:string)
                    n283 = case shown="Default" w457 {
                      tunnel: w456 -> [w458 w464]
                      frame "Time" {
                        n284 = local read "Parameter"() -> (w461:u16)
                        n285 = local read "Durations"() -> (w459:dbl[])
                        n286 = Replace Array Subset(array=w459, new element=w458, index=w461) -> (w460:dbl[])
                        n287 = local write "Durations"(w460) -> ()
                      }
                      frame Default {
                        w465 = u32 5 items=["Open", "Close", "Begin", "End", "Get", "Set"] ("Mode")
                        n288 = local read "Parameter"() -> (w463:u16)
                        n289 = local read "Item Function"() -> (w466:refnum<vi>)
                        n290 = Build Array(w464, w463) -> (w462:dbl[])
                        n291 = call-by-ref "?"(reference=w466, "In"=w462, "Mode"=w465) -> ()  [unwired: 1 in, 3 out]
                      }
                    }
                  }
                  frame #1 {
                    n292 = local write "Set"(FALSE ("Ready")) -> ()
                  }
                }
              }
            }
          }
          event "Device": Value Change {
            w472 = 2  # Ion Number
            n293 = event-data() -> ("NewVal"=w469:string)  [unwired: 1 in, 5 out]
            n294 = case shown="\"PMT\", Default" w469 {
              tunnel: [FALSE TRUE] -> w470
              tunnel: [1 260] -> w468
              frame "PMT", Default {
              }
              frame "CCD" {
              }
            }
            n295 = case shown="\"PMT\"" w469 {
              tunnel: [_ "c1+c2+c3+c4" "10*sin(x)^2"] -> w473
              frame Default {
              }
              frame "PMT" {
              }
              frame "Test" {
              }
            }
            n296 = local write ">"(w468) -> ()
            n297 = Decrement(x=w472) -> (x-1=w471:i32)
            n298 = for {
              N: w471 -> [_]
              tunnel: w470 -> [w476]
              i -> [w475]
              n299 = Increment(x=w475) -> (x+1=w474:i32)
              n300 = property on="Average Plot" class="WFChart (strict)"("Active Plot"=w474, "Plot.Visible?"=w476) -> ("DigDisps[]"=w477:refnum<vi>[])  [unwired: 2 in, 2 out]
              n301 = Index Array(array=w477, index=w474) -> (element=w478:refnum<vi>)
              n302 = property class="DigNum"(reference=w478, "Visible"=w476) -> ()  [unwired: 1 in, 2 out]
            }
            n303 = local write "Channel"(w473) -> ()
          }
          event Timeout {
            n304 = event-data() -> ()  [unwired: 1 in, 3 out]
            n305 = local read "Sweep"() -> (w487:bool)
            n306 = local read "Scan"() -> (w486:bool)
            n307 = Or(x=w487, y=w486) -> (x .or. y?=w485:bool)
            n308 = case shown="False" w485 {
              frame False {
              }
              frame True {
              }
            }
            n309 = Get Date/Time In Seconds() -> (seconds since 1Jan1904=w488:timestamp)
            n310 = Format Date/Time String(time format string (%c)="%Y/%m/%d %H:%M:%S", seconds (now)=w488) -> (date/time string=→"Clock":string)  [unwired: 1 in]
          }
          event "Protect": Value Change {
            n311 = event-data() -> ("NewVal"=w491:bool)  [unwired: 1 in, 5 out]
            n312 = case shown="True" w491 {
              frame False {
              }
              frame True {
                n313 = local read "Ion"() -> (w492:bool)
                n314 = property on="Ion" class="Bool (strict)"("Val(Sgnl)"=w492) -> ()  [unwired: 2 in, 2 out]
              }
            }
          }
          event "Start": Value Change {
            n315 = event-data() -> ("NewVal"=w493:dbl)  [unwired: 1 in, 5 out]
            n316 = flat-sequence {
              tunnel: w493 -> [w494]
              frame #0 {
                n317 = local write "Value"(w494) -> ()
              }
              frame #1 {
                n318 = property on="Set" class="Bool (strict)"("Val(Sgnl)"=TRUE ("Value (Signaling)")) -> ()  [unwired: 2 in, 2 out]
              }
            }
          }
          event "Sequencer": Value Change {
            n319 = event-data() -> ("NewVal"=w496:bool)  [unwired: 1 in, 4 out]
          }
          event "Send": Value Change {
            n320 = event-data() -> ("NewVal"=w498:bool)  [unwired: 1 in, 4 out]
            n321 = case shown="True" w498 {
              tunnel: w497 -> [_ w499]
              frame False {
              }
              frame True {
                n322 = flat-sequence {
                  tunnel: w499 -> [w500]
                  frame #0 {
                    n323 = local read "Period (ns)"() -> (w504:dbl)
                    n324 = local read "Durations"() -> (w502:dbl[])
                    n325 = local read "Repeats"() -> (w503:u32)
                    n326 = local read "States"() -> (w505:string[])
                    n327 = call "FPGAPackets.vi"("Repeats"=w503, "Period (ns)"=w504, "Durations"=w502, "States"=w505) -> ("Packets"=w501:string)  [unwired: 1 in, 1 out]
                    n328 = call "TxRS232.vi"("VISA resource name"=w500, "Data"=w501) -> ()
                  }
                  frame #1 {
                    n329 = local write "Send"(FALSE ("Send")) -> ()
                  }
                }
              }
            }
          }
        }
      }
      n330 = while {
        tunnel: w8 -> [w9]
        stop <- w10 stop-if-true
        n331 = event shown="[1] \"Scan\": Value Change" {
          selector: _ -> [_ _ _]
          dyn-events: _ -> [_ _ _]
          timeout: _ -> [_ _ _]
          tunnel: [_ _ w258] -> w10
          tunnel: w9 -> [_ w46 _]
          event "Cooling", "Pumping", "Detection", "Experiment": Value Change {
            n332 = event-data() -> ("CtlRef"=w12:refnum<vi>, "NewVal"=w11:bool)  [unwired: 1 in, 4 out]
            n333 = case shown="True" w11 {
              tunnel: w12 -> [_ w16]
              frame False {
              }
              frame True {
                n334 = flat-sequence {
                  tunnel: w16 -> [w18]
                  tunnel: [w18] -> w14
                  tunnel: w14 -> [w19]
                  tunnel: [w19] -> w13
                  tunnel: [w30] -> w15
                  tunnel: w13 -> [w28]
                  tunnel: w15 -> [w45]
                  frame #0 {
                    n335 = local write "Sweep"(FALSE ("Sweep")) -> ()
                  }
                  frame #1 {
                    n336 = while {
                      stop <- w21 continue-if-true
                      n337 = Wait (ms)(milliseconds to wait=u32 50) -> ()  [unwired: 1 out]
                      n338 = local read "Data"() -> (w21:bool)
                    }
                  }
                  frame #2 {
                    n339 = local read "Device"() -> (w24:string)
                    n340 = case shown="\"PMT\", Default" w24 {
                      tunnel: ["C" ("string") _] -> w22
                      frame "CCD" {
                      }
                      frame "PMT", Default {
                      }
                    }
                    n341 = property class="Bool (strict)"(reference=w28) -> (reference out=w30:refnum<vi>, "BoolText.Text"=w26:string)  [unwired: 1 in, 1 out]
                    n342 = Concatenate Strings(w26, w22, ".seq" ("string")) -> (w27:string)
                    n343 = Build Path(base path=path "E:/Data/Sequence", name or relative path=w27) -> (appended path=w25:path)
                    n344 = case shown="Default" w26 {
                      tunnel: w25 -> [w32 w34]
                      frame Default {
                        n345 = property on="Sequence File" class="Path"("Val(Sgnl)"=w32) -> ()  [unwired: 2 in, 2 out]
                      }
                      frame "Cooling", "Detection", "Pumping" {
                        n346 = flat-sequence {
                          tunnel: w34 -> [w36]
                          tunnel: [w36] -> w33
                          tunnel: w33 -> [w41]
                          frame #0 {
                            n347 = local read "Sequence File"() -> (w39:path)
                            n348 = Strip Path(path=w39) -> (name=w38:string)  [unwired: 1 out]
                            n349 = Search/Split String(string=w38, search string/char (-)=".") -> (substring before match=w35:string)  [unwired: 1 in, 2 out]
                            n350 = case shown="Default" w35 {
                              tunnel: w35 -> [_ w40]
                              frame "Cooling", "Detection", "Pumping" {
                              }
                              frame Default {
                                n351 = property on="Experiment" class="Bool (strict)"("BoolText.Text"=w40) -> ()  [unwired: 2 in, 2 out]
                              }
                            }
                          }
                          frame #1 {
                            n352 = property on="Sequence File" class="Path"("Val(Sgnl)"=w41) -> ()  [unwired: 2 in, 2 out]
                          }
                          frame #2 {
                            n353 = Wait (ms)(milliseconds to wait=u32 300) -> ()  [unwired: 1 out]
                          }
                          frame #3 {
                            n354 = property on="Sweep" class="Bool (strict)"("Val(Sgnl)"=TRUE ("Value (Signaling)")) -> ()  [unwired: 2 in, 2 out]
                          }
                        }
                      }
                    }
                  }
                  frame #3 {
                    n355 = property class="Bool (strict)"(reference=w45, "Value"=FALSE) -> ()  [unwired: 1 in, 2 out]
                  }
                }
              }
            }
          }
          event "Scan": Value Change {
            n356 = event-data() -> ("NewVal"=w47:bool)  [unwired: 1 in, 5 out]
            n357 = case shown="True" w47 {
              tunnel: w46 -> [w63 _]
              frame True {
                n358 = local read "Item"() -> (w65:string)
                n359 = Concatenate Strings(w65, "Scan-" ("string")) -> (w64:string)
                n360 = local read "Start"() -> (w74:dbl)
                n361 = flat-sequence {
                  tunnel: w64 -> [w80]
                  tunnel: w74 -> [w81]
                  tunnel: "Step" -> [w82]
                  tunnel: "End" -> [w83]
                  tunnel: w65 -> [w84]
                  tunnel: [w84] -> w59
                  tunnel: [w83] -> w57
                  tunnel: [w82] -> w55
                  tunnel: [w81] -> w53
                  tunnel: [w80] -> w51
                  tunnel: w63 -> [w79]
                  tunnel: [w78] -> w49
                  tunnel: w59 -> [w91]
                  tunnel: [w91] -> w58
                  tunnel: w57 -> [w90]
                  tunnel: [w90] -> w56
                  tunnel: w55 -> [w89]
                  tunnel: [w89] -> w54
                  tunnel: w53 -> [w88]
                  tunnel: [w88] -> w52
                  tunnel: w51 -> [w87]
                  tunnel: [w87] -> w50
                  tunnel: w49 -> [w86]
                  tunnel: [w86] -> w48
                  tunnel: [w109] -> w72
                  tunnel: [w98] -> w71
                  tunnel: [w103] -> w70
                  tunnel: [w102] -> w69
                  tunnel: [w101] -> w68
                  tunnel: [w100] -> w67
                  tunnel: w58 -> [w109]
                  tunnel: w56 -> [w106]
                  tunnel: w54 -> [w100]
                  tunnel: w52 -> [w101]
                  tunnel: w50 -> [w110]
                  tunnel: [w92] -> w61
                  tunnel: w48 -> [w92]
                  tunnel: [w149] -> w73
                  tunnel: w72 -> [w149]
                  tunnel: w71 -> [w155]
                  tunnel: w70 -> [w154]
                  tunnel: w69 -> [w153]
                  tunnel: w68 -> [w152]
                  tunnel: w67 -> [w151]
                  tunnel: [w150] -> w66
                  tunnel: [w148] -> w62
                  tunnel: w61 -> [w148]
                  tunnel: w73 -> [w252]
                  tunnel: w66 -> [w247]
                  tunnel: w62 -> [w245]
                  tunnel: [w245] -> w60
                  tunnel: w60 -> [w257]
                  frame #0 {
                    n362 = call "SequencerInitRS232.vi"("VISA resource name"=w79) -> ("reference out"=w78:refnum<visa-resource-name>)  [unwired: 1 out]
                  }
                  frame #1 {
                    n363 = Wait (ms)(milliseconds to wait=u32 200) -> ()  [unwired: 1 out]
                  }
                  frame #2 {
                    w114 = "\r\n"
                    n364 = Subtract(x=w106, y=w101) -> (x-y=w105:dbl)
                    n365 = local read "Parameter"() -> (w97:u16)
                    n366 = property on="Average Plot" class="WFChart (strict)"() -> ("History Data"=w96:cluster{dbl, dbl}[])  [unwired: 2 in, 2 out]
                    n367 = Divide(x=w105, y=w100) -> (x/y=w104:dbl)
                    n368 = case shown="Default" w109 {
                      tunnel: ["us" ("string") w137] -> w108
                      tunnel: [w128 w145] -> w107
                      tunnel: w97 -> [w124 w141]
                      frame "Time" {
                        n369 = local read "Durations"() -> (w135:dbl[])
                        n370 = local write "Durations Backup"(w135) -> ()
                        n371 = local read "Chapter (us)"() -> (w133:string)
                        n372 = local read "Sequence"() -> (w132:string)
                        n373 = call "SaveSequenceString.vi"("Sequence"=w132, "Chapter"=w133) -> ("Sequence String"=w130:string)
                        n374 = Number To Decimal String(number=w124) -> (decimal integer string=w126:string)  [unwired: 1 in]
                        n375 = Concatenate Strings("Sequence=\n{\n" ("string"), w130, "\n}\n" ("string"), "Index=" ("string"), w126, "\r\n") -> (w128:string)
                      }
                      frame Default {
                        w143 = u32 2 items=["Open", "Close", "Begin", "End", "Get", "Set"] ("Mode")
                        n376 = local read "Item Function"() -> (w142:refnum<vi>)
                        n377 = call-by-ref "?"(reference=w142, "In"=w141, "Mode"=w143) -> ("Out"=w140:variant)  [unwired: 1 in, 2 out]
                        n378 = Variant To Data(type=string[] [] ("Strings []"), Variant=w140) -> (data=w138:string[])  [unwired: 1 in, 1 out]
                        n379 = property on="Parameter" class="Ring (strict)"() -> ("RingText.Text"=w144:string)  [unwired: 2 in, 2 out]
                        n380 = Index Array(array=w138) -> (element #1=w137:string, element #2=w136:string)  [unwired: 2 in]
                        n381 = Concatenate Strings("Parameter=" ("string"), w144, "\r\n", w136) -> (w145:string)
                      }
                    }
                    n382 = Round Toward -Infinity(1:w104) -> (0:w99:dbl)
                    n383 = Array Subset(array=w96, length=0) -> (w94:cluster{dbl, dbl}[])  [unwired: 1 in]
                    n384 = property on="Average Plot" class="WFChart (strict)"("History Data"=w94, "XScale.Multiplier"=w100, "XScale.Offset"=w101, "XScale.Maximum"=w106) -> ()  [unwired: 2 in, 2 out]
                    n385 = To Unsigned Long Integer(number=w99) -> (unsigned 32bit integer=w98:u32)
                    n386 = call <vilib>:"Space Constant.vi"() -> ("String"=w113:string)
                    n387 = Concatenate Strings(w113, w108) -> (w103:string)
                    n388 = Number To Fractional String(number=w101) -> (F-format string=w121:string)  [unwired: 3 in]
                    n389 = Number To Fractional String(number=w106) -> (F-format string=w119:string)  [unwired: 3 in]
                    n390 = Number To Fractional String(number=w100) -> (F-format string=w117:string)  [unwired: 3 in]
                    n391 = call "NewData.vi"("Prefix"=w110, "data location"=path "E:/Data") -> ("data file name"=w111:string, "data file refnum"=w112:refnum<file>)  [unwired: 1 in]
                    n392 = local write "data file"(w111) -> ()
                    n393 = Concatenate Strings(w107, "Start=" ("string"), w121, w103, w114, "End=" ("string"), w119, w103, w114, "Step=" ("string"), w117, w103, w114, "Counts=" ("string"), w114, "{" ("string"), w114) -> (w122:string)
                    n394 = Write to Text File(file (use dialog)=w112, text=w122) -> (refnum out=w102:refnum<file>)  [unwired: 2 in, 2 out]
                  }
                  frame #3 {
                    n395 = while {
                      tunnel: w155 -> [w166]
                      tunnel: w154 -> [w162]
                      tunnel: w153 -> [w161]
                      shift-right: [w158] -> _
                      shift-left: w152 -> [w157]
                      tunnel: w151 -> [w160]
                      tunnel: [w159] -> w150
                      tunnel: w148 -> [w156]
                      i -> [w167]
                      stop <- w163 continue-if-true
                      n396 = flat-sequence {
                        tunnel: w157 -> [w168]
                        tunnel: w156 -> [w171]
                        tunnel: w162 -> [w233]
                        tunnel: w161 -> [w231]
                        tunnel: [w230] -> w159
                        tunnel: w157 -> [w229]
                        frame #0 {
                          n397 = local write "Value"(w168) -> ()
                        }
                        frame #1 {
                          n398 = property on="Set" class="Bool (strict)"("Val(Sgnl)"=TRUE ("Ready")) -> ()  [unwired: 2 in, 2 out]
                        }
                        frame #2 {
                          n399 = while {
                            stop <- w170 continue-if-true
                            n400 = local read "Set"() -> (w170:bool)
                          }
                        }
                        frame #3 {
                          n401 = while {
                            tunnel: w171 -> [w178]
                            stop <- w173 stop-if-true
                            n402 = flat-sequence {
                              tunnel: w178 -> [w182]
                              tunnel: [w182] -> w177
                              tunnel: [w181] -> w176
                              tunnel: w177 -> [w190]
                              tunnel: w176 -> [w189]
                              tunnel: [w187] -> w175
                              tunnel: [w217] -> w174
                              tunnel: w175 -> [w217]
                              tunnel: [w216] -> w172
                              frame #0 {
                                n403 = property on="Data" class="Bool (strict)"("Val(Sgnl)"=TRUE ("Value (Signaling)")) -> ()  [unwired: 2 in, 2 out]
                              }
                              frame #1 {
                                n404 = while {
                                stop <- w180 continue-if-true
                                n405 = local read "Data"() -> (w180:bool)
                                }
                              }
                              frame #2 {
                                w181 = u32 100 ("Repeats")
                                n406 = local read "Period (ns)"() -> (w186:dbl)
                                n407 = call "FPGAPackets.vi"("Repeats"=w181, "Period (ns)"=w186, "Durations"=dbl[] [1000.0, 1.0, 1.0, 10.0], "States"=string[] ["00000000000000000000000000001111", "00000000000000000000000000000000", "00000000000000000000000000010000", "10000000000000000000000000000000"]) -> ("Packets"=w183:string)  [unwired: 1 in, 1 out]
                                n408 = call "TxRS232.vi"("VISA resource name"=w182, "Data"=w183) -> ()
                              }
                              frame #3 {
                                n409 = local read "Device"() -> (w188:string)
                                n410 = case shown="\"PMT\", Default" w188 {
                                tunnel: w190 -> [_ w194]
                                tunnel: w189 -> [_ w204]
                                tunnel: [TRUE w195] -> w187
                                frame "CCD" {
                                }
                                frame "PMT", Default {
                                n411 = Multiply(x=w204, y=u32 4) -> (x*y=w203:u32)
                                n412 = Multiply(x=w203, y=3 ("Bytes To Read")) -> (x*y=w193:u32)
                                n413 = VISA Read(VISA resource name=w194, byte count=w193) -> (read buffer=w192:string)  [unwired: 1 in, 3 out]
                                n414 = for {
                                N: w203 -> [_]
                                tunnel: w192 -> [w215]
                                tunnel: [w206] -> w201 mode=indexing
                                i -> [w209]
                                w208 = 3 ("length (rest)")
                                n415 = Multiply(x=w209, y=w208) -> (x*y=w207:i32)
                                n416 = String Subset(string=w215, offset (0)=w207, length (rest)=w208) -> (substring=w210:string)
                                n417 = Concatenate Strings("\u0000" ("string"), w210) -> (w214:string)
                                n418 = To Unsigned Long Integer(number=u32 0) -> (unsigned 32bit integer=w211:u32)
                                n419 = Type Cast(type=w211, x=w214) -> (*(type *) &x=w206:u32)
                                }
                                n420 = Decimate 1D Array(w201) -> (w199:u32[])  [unwired: 3 out]
                                n421 = Add Array Elements(numeric array=w199) -> (sum=w200:u32)
                                n422 = Array Size(array=w199) -> (size(s)=w198:i32)
                                n423 = Divide(x=w200, y=w198) -> (x/y=w197:dbl)
                                n424 = Greater?(x=w197, y=2.0) -> (0:w195:bool)
                                }
                                }
                              }
                              frame #4 {
                                n425 = case shown="False" w217 {
                                selector: w217 -> [w219 w228]
                                tunnel: [w218 FALSE] -> w216
                                frame False {
                                n426 = flat-sequence {
                                tunnel: w219 -> [w220]
                                tunnel: [w221] -> w218
                                frame #0 {
                                n427 = property on="Ion" class="Bool (strict)"("Val(Sgnl)"=w220) -> ()  [unwired: 2 in, 2 out]
                                }
                                frame #1 {
                                n428 = while {
                                tunnel: [w222] -> w221
                                stop <- w223 stop-if-true
                                n429 = local read "Scan"() -> (w224:bool)
                                n430 = Wait (ms)(milliseconds to wait=u32 1000) -> ()  [unwired: 1 out]
                                n431 = Not(x=w224) -> (.not. x?=w222:bool)
                                n432 = local read "Ion"() -> (w225:bool)
                                n433 = Or(x=w225, y=w222) -> (x .or. y?=w223:bool)
                                }
                                }
                                }
                                }
                                frame True {
                                n434 = local write "Ion"(w228) -> ()
                                }
                                }
                              }
                            }
                            n435 = Or(x=w174, y=w172) -> (x .or. y?=w173:bool)
                          }
                        }
                        frame #4 {
                          n436 = Number To Fractional String(number=w229) -> (F-format string=w239:string)  [unwired: 3 in]
                          n437 = local read "Counts"() -> (w234:u32[])
                          n438 = Concatenate Strings(w239, w233, "," ("string")) -> (w238:string)
                          n439 = for {
                            tunnel: w234 -> [w244] mode=indexing
                            shift-right: [w242] -> w235
                            shift-left: w238 -> [w241]
                            n440 = Number To Decimal String(number=w244) -> (decimal integer string=w243:string)  [unwired: 1 in]
                            n441 = call <vilib>:"Space Constant.vi"() -> ("String"=w240:string)
                            n442 = Concatenate Strings(w241, w240, w243) -> (w242:string)
                          }
                          n443 = Concatenate Strings(w235, "\r\n") -> (w236:string)
                          n444 = Write to Text File(file (use dialog)=w231, text=w236) -> (refnum out=w230:refnum<file>)  [unwired: 2 in, 2 out]
                        }
                      }
                      n445 = Add(x=w157, y=w160) -> (x+y=w158:dbl)
                      n446 = Less?(x=w167, y=w166) -> (x < y?=w165:bool)
                      n447 = local read "Scan"() -> (w164:bool)
                      n448 = And(x=w165, y=w164) -> (x .and. y?=w163:bool)
                    }
                  }
                  frame #4 {
                    n449 = case shown="\"Time\"" w252 {
                      frame "Time" {
                        n450 = local read "Durations Backup"() -> (w253:dbl[])
                        n451 = local write "Durations"(w253) -> ()
                      }
                      frame Default {
                        w256 = u32 3 items=["Open", "Close", "Begin", "End", "Get", "Set"] ("Mode")
                        n452 = local read "Item Function"() -> (w255:refnum<vi>)
                        n453 = local read "Parameter"() -> (w254:u16)
                        n454 = call-by-ref "?"(reference=w255, "In"=w254, "Mode"=w256) -> ()  [unwired: 1 in, 3 out]
                      }
                    }
                    n455 = local write "Scan"(FALSE ("Scan")) -> ()
                    n456 = Concatenate Strings("}" ("string"), "\r\n") -> (w248:string)
                    n457 = Write to Text File(file (use dialog)=w247, text=w248) -> (refnum out=w251:refnum<file>)  [unwired: 2 in, 2 out]
                    n458 = Close File(refnum=w251) -> ()  [unwired: 1 in, 2 out]
                  }
                  frame #5 {
                    n459 = VISA Close(VISA resource name=w257) -> ()  [unwired: 1 in, 1 out]
                  }
                }
              }
              frame False, Default {
              }
            }
          }
          event "Sequencer": Value Change {
            n460 = event-data() -> ("NewVal"=w259:bool)  [unwired: 1 in, 5 out]
            n461 = flat-sequence {
              tunnel: [w261] -> w260
              tunnel: w259 -> [w261]
              tunnel: w260 -> [w264]
              tunnel: [w264] -> w258
              frame #0 {
                n462 = local write "Sweep"(FALSE ("Sweep")) -> ()
                n463 = local write "Scan"(FALSE ("Scan")) -> ()
              }
              frame #1 {
                n464 = property on="Data" class="Bool (strict)"("Val(Sgnl)"=FALSE ("Value (Signaling)")) -> ()  [unwired: 2 in, 2 out]
              }
            }
          }
        }
      }
    }
    frame #2 {
      n465 = local read "Port"() -> (w727:refnum<visa-resource-name>)
      n466 = VISA Close(VISA resource name=w727) -> ()  [unwired: 1 in, 1 out]
    }
  }
